vi "State Machine - Send Message to Process.vi"(5 "Data":variant, 6 "Front?":bool, 7 "State":string, 8 "error in (no error)":errorcluster, 11 "Process Name":string) -> (0 "error out":errorcluster)   [LabVIEW 2015, in "State Machine.lvlib"]
uses:
  State Machine.lvlib
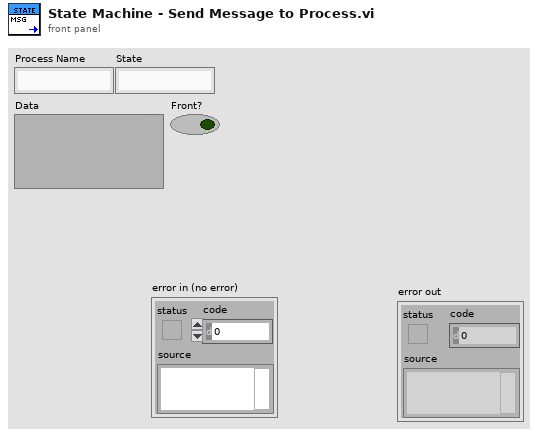
[diagram p1: front panel]
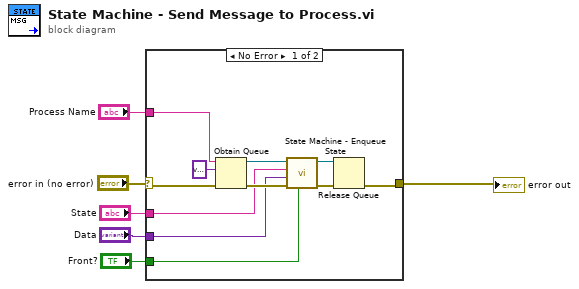
[diagram p0: block diagram]
diagram:
  n1 = case shown="No Error" "error in (no error)" {
    selector: "error in (no error)" -> [w13 w18]
    tunnel: [w12 w18] -> w6
    tunnel: "Process Name" -> [w11 _]
    tunnel: "Data" -> [w8 _]
    tunnel: "State" -> [w10 _]
    tunnel: "Front?" -> [w7 _]
    frame No Error {
      n2 = Obtain Queue(name (unnamed)=w11, element data type=variant, error in (no error)=w13) -> (queue out=w16:refnum<queue>, error out=w17:errorcluster)  [unwired: 2 in, 1 out]
      n3 = call "State Machine - Enqueue State.vi"("Front?"=w7, "error in (no error)"=w17, "Data"=w8, "State"=w10, "Queue In"=w16) -> ("error out"=w15:errorcluster, "Queue Out"=w14:refnum<queue>)  [unwired: 5 in]
      n4 = Release Queue(queue=w14, error in (no error)=w15) -> (error out=w12:errorcluster)  [unwired: 1 in, 2 out]
    }
    frame Error {
    }
  }
  "error out" <- w6
